vi "CorrectDistance.vi"(3 "CenterPoint":dbl=24.0 format="%#_13g", 5 "Distance":dbl=56.0762 format="%#_13g") -> (19 "In Range?":bool, 21 "Right Motor":dbl=0.5 format="%#_13g", 22 "Left Motor":dbl=0.5 format="%#_13g")   [LabVIEW 2016]
panel:
  in  "Bad Value Count":i32=4
  in  "Speed":dbl=0.5 format="%#_13g"
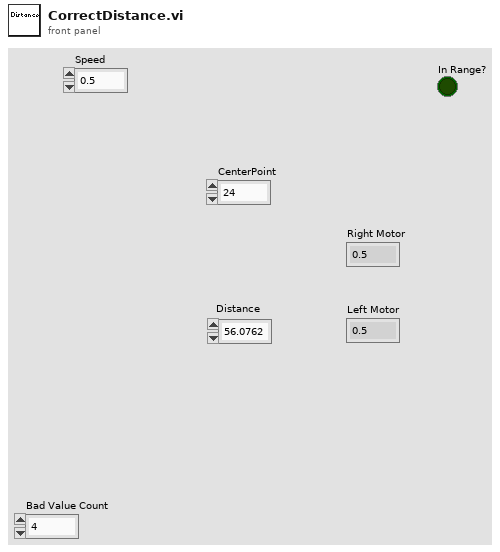
[diagram p1: front panel]
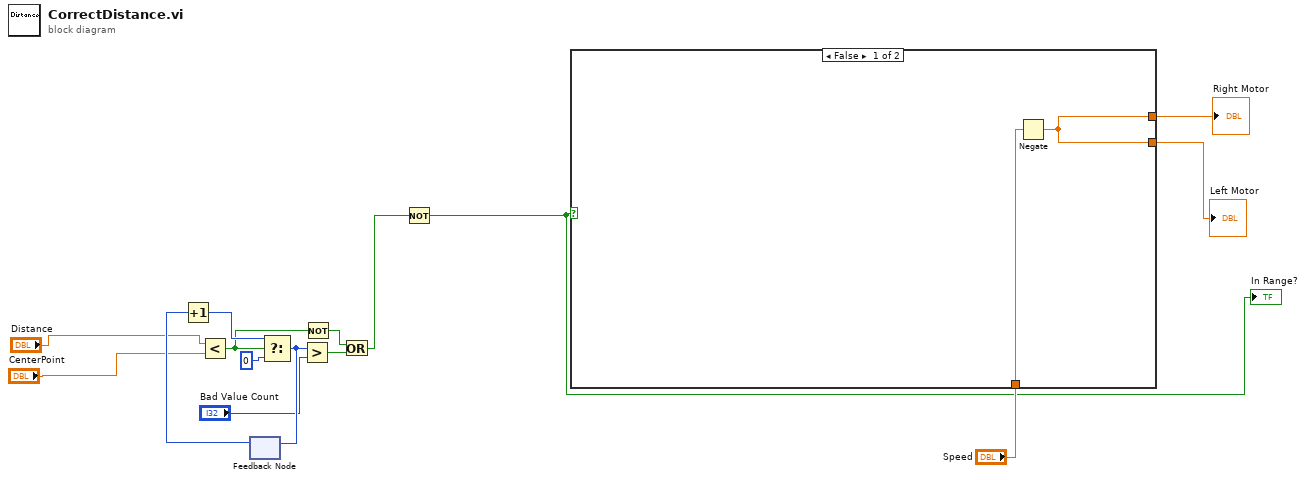
[diagram p0: block diagram]
diagram:
  n1 = Less?(x="Distance", y="CenterPoint") -> (x < y?=w6:bool)
  n2 = feedback #1() -> (w10:i32)  [unwired: 1 in]
  n3 = Increment(x=w10) -> (x+1=w11:i32)
  n4 = Select(t=w11, s=w6, f=0) -> (s? t:f=w9:i32)
  n5 = feedback-in #1(w9) -> ()
  n6 = Greater?(x=w9, y="Bad Value Count") -> (0:w7:bool)
  n7 = Not(x=w6) -> (.not. x?=w5:bool)
  n8 = Or(x=w5, y=w7) -> (x .or. y?=w2:bool)
  n9 = Not(x=w2) -> (.not. x?=w1:bool)
  "In Range?" <- w1
  n10 = case shown="False" w1 {
    tunnel: [w16 w18] -> w15
    tunnel: [w16 w18] -> w14
    tunnel: "Speed" -> [w17 w18]
    frame False {
      n11 = Negate(x=w17) -> (-x=w16:dbl)
    }
    frame True {
    }
  }
  "Right Motor" <- w15
  "Left Motor" <- w14
